vi "Acquire TCP AI.vi"(0 "connection ID":refnum<k5>, 5 "channels":i32, 11 "error in":errorcluster) -> (4 "connection ID out":refnum<k5>, 6 "voltage data":sgl[][](array[numeric]) format="%.2f", 8 "samples":u32, 10 "data array":T1[](array[typedef]) {"seconds since 1904" format="%.2f"; "voltage data" format="%.4f"}, 15 "error out":errorcluster)   [LabVIEW 2019]
doc: "This VI is usually used in a while loop to acquire data continuously from the data server. The number of data scans acquired is variable.\n\nInputs\n\nConnection ID in - TCP connection\n\nChannels - The number of channels being monitored. This is required to determine the size of the TCP data packet. The size of the data packet is 20 + 4i bytes where i is the number of channels being monitored.\n\nError in - \n\nOutputs\n\nConnection ID out - TCP connection\n\nVoltage data - Two dimensional array of data received from the data server. The first dimension is the scans and the second dimension is the channels.\n\nSamples - Number of scans that were received (size of the first dimension of the voltage data array.\n\nData array -Array of data clusters sent from the data server to the client.\n\nElements \n\nVoltage data - a one dimensional array of data received from the data server.\n\nArbitrary time (s) - The time since the data server began monitoring the channels. (Not the time since the client began monitoring). \n\nScan backlog out - the backlog of the data server data acquisition process. The scan backlog should be zero or very close to zero. If it isn't it suggests that the data rate and/or number of clients is too high.\n\nArbitrary scans - Number of scans made by the data server since the data server began monitoring channels.\n\n\nError out - \n\n\nCreated by Monroe Weber-Shirk\nCornell University\nmw24@cornell.edu\nJanuary 2000"
uses:
  DataServer/data send.ctl
panel:
  in  "data":T1={"voltage data"=[0.0, 0.0, 0.0, 0.0, 0.0, 0.0048828125, 0.0, 0.0, 0.0, 0.0, 0.0024414062, 0.0024414062, 0.0, 0.0, 0.0, 0.0024414062, 0.0, 0.0048828125, 0.0024414062, 0.0048828125, 0.0, 0.0024414062, 0.0024414062, 0.0048828125, 0.01953125, 0.017089844, 0.012207031, 0.0146484375, 0.0146484375, 0.0146484375, 0.01953125, 0.009765625], "scan backlog"=0, "seconds since 1904"=0.0, "arbitrary scans"=0} {"seconds since 1904" format="%.2f"; "voltage data" format="%.4f"}
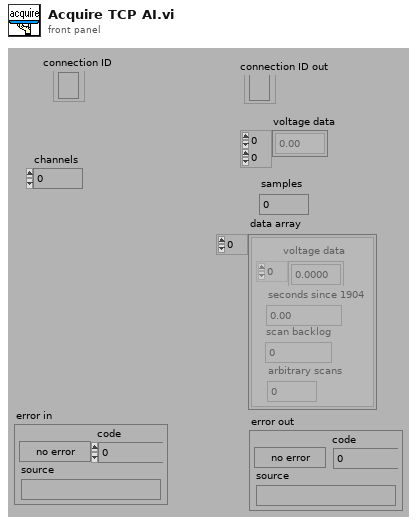
[diagram p1: front panel]
types:
  T1 = typedef "data send.ctl" = cluster{"voltage data":sgl[], "scan backlog":u32, "seconds since 1904":dbl, "arbitrary scans":i32}
  T2 = cluster{"voltage data":sgl[], "scan backlog out":u32, "arbitrary time (s)":dbl, "arbitrary scans":i32}[]
  T3 = enum16{"Standard", "Buffered", "CRLF", "Immediate"}
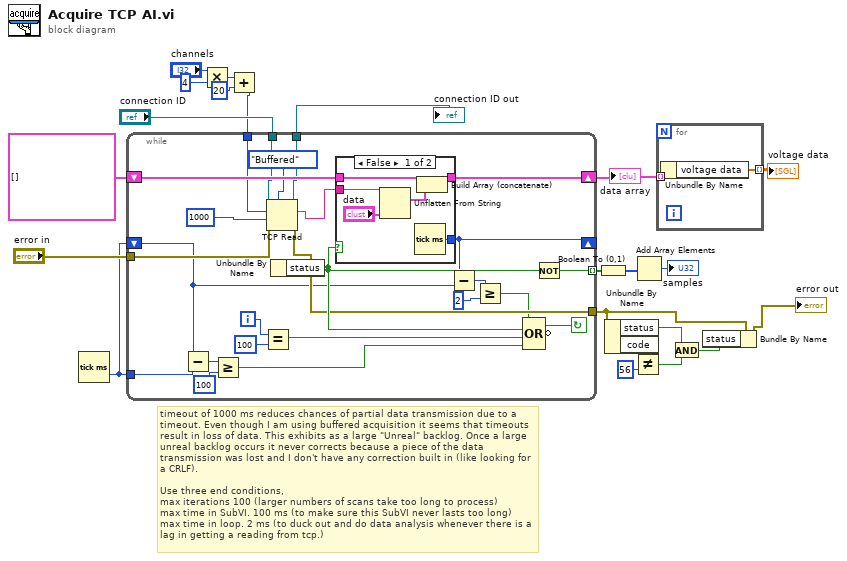
[diagram p0: block diagram]
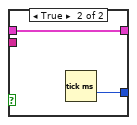
[diagram p2: hidden frame]
diagram:
  # "timeout of 1000 ms reduces chances of partial data transmission due to a timeout. Even though I am using buffered acquisition it seems that timeouts result in loss of data. This exhibits as a large \"Unreal\" backlog. Once a large unreal backlog occurs it never corrects because a piece of the data transmission was lost and I don't have any correction built in (like looking for a CRLF).\n\nUse three end conditions, \nmax iterations 100 (larger numbers of scans take too long to process)\nmax time in SubVI. 100 ms (to make sure this SubVI never lasts too long)\nmax time in loop. 2 ms (to duck out and do data analysis whenever there is a lag in getting a reading from tcp.)"
  n1 = Tick Count (ms)() -> (millisecond timer value=w2:u32)
  n2 = Multiply(x="channels", y=4) -> (x*y=w4:i32)
  n3 = Add(x=w4, y=20) -> (x+y=w3:i32)
  n4 = while {
    shift-left: w2 -> [w27]
    shift-right: [w26] -> _
    tunnel: w2 -> [w31]
    tunnel: w3 -> [w33]
    tunnel: [w45] -> w19 mode=indexing
    shift-left: T2 [] -> [w47]
    shift-right: [w46] -> w9
    tunnel: [w35] -> w16
    tunnel: "connection ID" -> [w38]
    tunnel: [w37] -> w21
    tunnel: "error in" -> [w40]
    i -> [w42]
    stop <- w43 continue-if-true
    n5 = Subtract(x=w27, y=w31) -> (x-y=w30:u32)
    n6 = Greater Or Equal?(x=w30, y=u32 100) -> (x >= y?=w28:bool)
    n7 = Equal?(x=w42, y=100) -> (x = y?=w41:bool)
    n8 = TCP Read(connection ID=w38, bytes to read=w33, error in (no error)=w40, 7:T3."Buffered" ("mode (standard)"), 9:1000) -> (connection ID out=w37:refnum<k5>, data out=w36:string, error out=w35:errorcluster)
    n9 = Unbundle By Name(w35) -> ("status"=w44:bool)
    n10 = case shown="False" w44 {
      tunnel: w47 -> [w53 w55]
      tunnel: [w52 w55] -> w46
      tunnel: w36 -> [w49 _]
      tunnel: [w48 w54] -> w26
      frame False {
        n11 = Unflatten From String(type="data", binary string=w49) -> (value=w50:T1)  [unwired: 3 in, 2 out]
        n12 = Tick Count (ms)() -> (millisecond timer value=w48:u32)
        n13 = Build Array (concatenate)(w53, w50) -> (w52:T1[])
      }
      frame True {
        n14 = Tick Count (ms)() -> (millisecond timer value=w54:u32)
      }
    }
    n15 = Subtract(x=w26, y=w27) -> (x-y=w25:u32)
    n16 = Greater Or Equal?(x=w25, y=u32 2) -> (x >= y?=w23:bool)
    n17 = Compound Arithmetic op=OR(w23, w44, w41, w28) -> (invert w43:bool)
    n18 = Not(x=w44) -> (.not. x?=w45:bool)
  }
  "connection ID out" <- w21
  "data array" <- w9
  n19 = Boolean To (0,1)(Boolean=w19) -> (0, 1=w18:i16[])
  n20 = Unbundle By Name(w16) -> ("status"=w13:bool, "code"=w14:i32)
  n21 = Not Equal?(x=w14, y=56) -> (x != y?=w12:bool)
  n22 = Add Array Elements(numeric array=w18) -> (sum=→"samples":i16)
  n23 = for {
    tunnel: w9 -> [w57] mode=indexing
    tunnel: [w56] -> w8 mode=indexing
    n24 = Unbundle By Name(w57) -> ("voltage data"=w56:sgl[])
  }
  "voltage data" <- w8
  n25 = And(x=w13, y=w12) -> (x .and. y?=w11:bool)
  n26 = Bundle By Name(cluster=w16, "status"=w11) -> (→"error out":errorcluster)
